vi "TSM DCPower Close Sessions.vi"(0 "TSM context":T1) -> (15 "error out":errorcluster)   [LabVIEW 2020]
uses:
  <vilib>/NI_TestStand_SemiconductorModule/NI_TestStand_Semiconductor_Module.lvlibp/PinMap/General/SemiconductorModuleContext.ctl
  <vilib>/NI_TestStand_SemiconductorModule/NI_TestStand_Semiconductor_Module.lvlibp
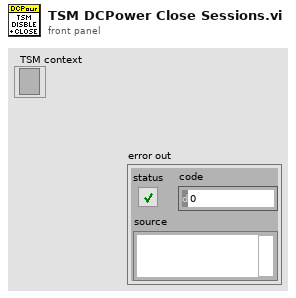
[diagram p1: front panel]
types:
  T1 = typedef "NI_TestStand_Semiconductor_Module.lvlibp/SemiconductorModuleContext.ctl" = refnum<k7>
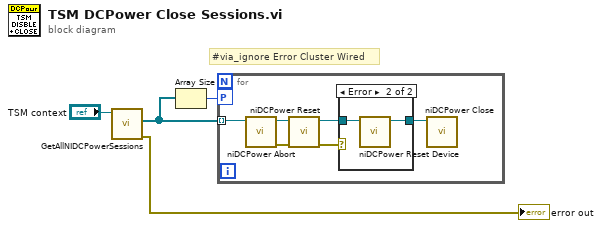
[diagram p0: block diagram]
diagram:
  # "#via_ignore Error Cluster Wired"
  n1 = call <vilib>:"GetAllNIDCPowerSessions.vi"("Semiconductor Module Context"="TSM context") -> ("error out"=→"error out":errorcluster, "Instrument Sessions"=w2:refnum<k15>[])  [unwired: 8 in, 1 out]
  n2 = Array Size(array=w2) -> (size(s)=w3:i32)
  n3 = for {
    workers-P: w3 -> [_]
    tunnel: w2 -> [w10] mode=indexing
    n4 = call <instrlib>:"niDCPower Abort.vi"("instrument handle"=w10) -> ("error out"=w7:errorcluster, "instrument handle out"=w9:refnum<k15>)  [unwired: 9 in]
    n5 = call <instrlib>:"niDCPower Reset.vi"("error in (no error)"=w7, "instrument handle"=w9) -> ("error out"=w5:errorcluster, "instrument handle out"=w8:refnum<k15>)  [unwired: 8 in]
    n6 = case shown="Error" w5 {
      tunnel: w8 -> [w11 w13]
      tunnel: [w11 w12] -> w6
      frame No Error {
      }
      frame Error {
        n7 = call <instrlib>:"niDCPower Reset Device.vi"("instrument handle"=w13) -> ("instrument handle out"=w12:refnum<k15>)  [unwired: 9 in, 1 out]
      }
    }
    n8 = call <instrlib>:"niDCPower Close.vi"("instrument handle"=w6) -> ()  [unwired: 10 in, 1 out]
  }
